vi "GenerateNewFilename.vi"(9 "Postfix":string="_info.txt", 10 "expname":string="exp0", 11 "Basepath":path=path "D:/labview/jelmer/labview tmp/traces") -> (3 "expname (out)":string)   [LabVIEW 2011]
uses:
  <vilib>/regexp/Match Regular Expression.xnode
panel:
  out "checking path..":string
  out "num":i32
  out "Output":string
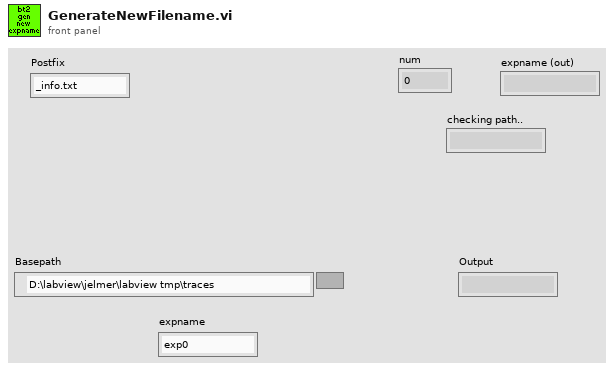
[diagram p1: front panel]
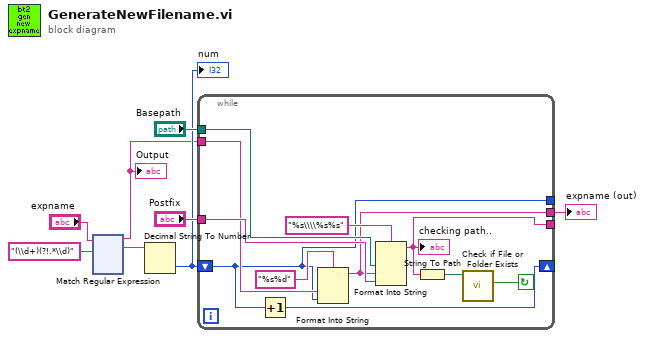
[diagram p0: block diagram]
diagram:
  n1 = xnode "Match Regular Expression"("input string"="expname", "regular expression"="(\\d+)(?!.*\\d)") -> ("before match"=w2:string, "whole match"=w6:string)  [unwired: 4 in, 3 out]
  "Output" <- w2
  n2 = Decimal String To Number(string=w6) -> (number=w3:i32)  [unwired: 2 in, 1 out]
  "num" <- w3
  n3 = while {
    tunnel: "Basepath" -> [w18]
    tunnel: "Postfix" -> [w17]
    tunnel: [w11] -> _
    shift-right: [w14] -> _
    shift-left: w3 -> [w13]
    tunnel: w2 -> [w15]
    tunnel: [w13] -> _
    tunnel: [w12] -> w1
    stop <- w9 continue-if-true
    n4 = Increment(x=w13) -> (x+1=w14:i32)
    n5 = Format Into String(format string="%s%d", w15, w13) -> (resulting string=w12:string)  [unwired: 2 in, 1 out]
    n6 = Format Into String(format string="%s\\\\%s%s", w18, w12, w17) -> (resulting string=w11:string)  [unwired: 2 in, 1 out]
    "checking path.." <- w11
    n7 = String To Path(string=w11) -> (path=w10:path)
    n8 = call <vilib>:"Check if File or Folder Exists.vi"("path"=w10) -> ("file or folder exists?"=w9:bool)  [unwired: 8 in, 2 out]
  }
  "expname (out)" <- w1
